vi "CTRL XY Movement.vi"(6 "Position in":T2, 8 "error in":errorcluster, 9 "Current Axis Info In":T1, 10 "Previous Axis Info In":T1, 11 "Ref In":refnum<vi>) -> (0 "error out":errorcluster, 2 "Position out":T2)   [LabVIEW 2012]
doc: "This VI will calculate new coordinates for an object and move it there."
uses:
  <vilib>/Utility/miscctls.llb/LVPositionTypeDef.ctl
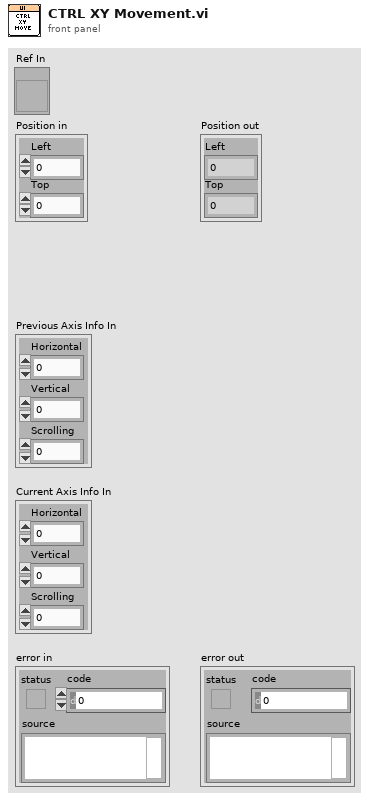
[diagram p1: front panel]
types:
  T1 = cluster{"Horizontal":i32, "Vertical":i32, "Scrolling":i32}
  T2 = typedef "LVPositionTypeDef.ctl" = cluster{"Left":i32, "Top":i32}
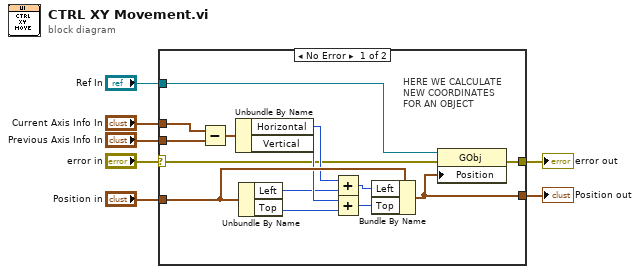
[diagram p0: block diagram]
diagram:
  n1 = case shown="No Error" "error in" {
    selector: "error in" -> [w8 w22]
    tunnel: [w20 _] -> w7
    tunnel: [w19 w22] -> w6
    tunnel: "Current Axis Info In" -> [w18 _]
    tunnel: "Position in" -> [w15 _]
    tunnel: "Previous Axis Info In" -> [w10 _]
    tunnel: "Ref In" -> [w9 _]
    frame No Error {
      # "HERE WE CALCULATE NEW COORDINATES FOR AN OBJECT"
      n2 = Subtract(x=w18, y=w10) -> (x-y=w21:T1)
      n3 = Unbundle By Name(w21) -> ("Horizontal"=w11:i32, "Vertical"=w13:i32)
      n4 = Unbundle By Name(w15) -> ("Left"=w12:i32, "Top"=w14:i32)
      n5 = Add(x=w11, y=w12) -> (x+y=w16:i32)
      n6 = Add(x=w13, y=w14) -> (x+y=w17:i32)
      n7 = Bundle By Name(cluster=w15, "Left"=w16, "Top"=w17) -> (w20:T2)
      n8 = property class="GObj"(reference=w9, error in=w8, "Position"=w20) -> (error out=w19:errorcluster)  [unwired: 1 out]
    }
    frame Error {
      # "ERROR OCCURED"
    }
  }
  "Position out" <- w7
  "error out" <- w6
